vi "Write DIO Bank States.vi"(5 "DIO Line Config":T2=[FALSE, FALSE, FALSE, FALSE, FALSE, FALSE, FALSE, FALSE], 6 "Output Cache in":u16, 7 "Logic Threshold (%)":u8, 8 "error in (no error)":errorcluster, 9 "Chip Address (A2 A1 A0)":T3 max=7, 10 "Slot #":T1 max=15, 11 "Rack #":u8) -> (0 "error out":errorcluster, 3 "FIFO SPI Message":u64 format="%b", 4 "Output Cache out":u16)   [LabVIEW 2014, in "SLSC configuration Shared.lvlib"]
uses:
  SLSC configuration Shared.lvlib
  MCP23S17/Chip Address.ctl
  DIO Line Config.ctl
  SPI Utility/Slot #.ctl
  MCP23S17/Write Digital All Pins.vi
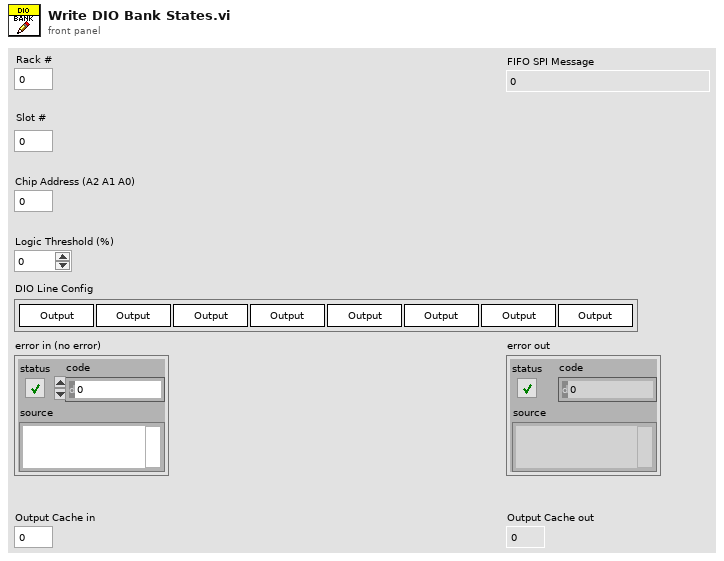
[diagram p1: front panel]
types:
  T1 = typedef "SLSC configuration Shared.lvlib/Slot #.ctl" = u8
  T2 = typedef "SLSC configuration Shared.lvlib/DIO Line Config.ctl" = bool[]
  T3 = typedef "SLSC configuration Shared.lvlib/Chip Address.ctl" = u8
  T4 = typedef "SLSC configuration Shared.lvlib/SPI Command.ctl" = cluster{"SPI Command":u32, "Transfer Length":u8}
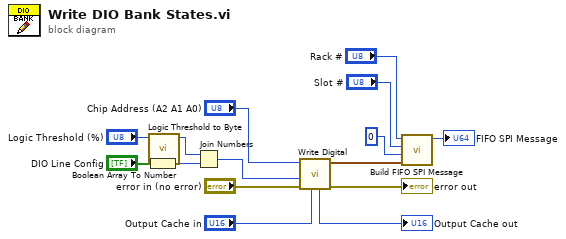
[diagram p0: block diagram]
diagram:
  n1 = Boolean Array To Number(Boolean array="DIO Line Config") -> (number=w11:u8)
  n2 = call "Logic Threshold to Byte.vi"("Logic Threshold (%)"="Logic Threshold (%)") -> ("Threshold Byte"=w12:u8)  [unwired: 10 in]
  n3 = Join Numbers(hi=w12, lo=w11) -> ((hi.lo)=w10:u16)
  n4 = call-poly "Write Digital.vi"("Output Cache in"="Output Cache in", "error in (no error)"="error in (no error)", "Value"=w10, "Chip Address (A2 A1 A0)"="Chip Address (A2 A1 A0)") -> ("error out"=→"error out":errorcluster, "SPI Command"=w6:T4, "Output Cache out"=→"Output Cache out":u16)  [unwired: 5 in]
  n5 = call "Build FIFO SPI Message.vi"("SPI Command"=w6, "Chip Select"=u8 0, "Slot #"="Slot #", "Rack #"="Rack #") -> ("FIFO SPI Message"=→"FIFO SPI Message":u64)  [unwired: 7 in]
